vi "Send Host Stream Command Start.vi"(6 "Project Folder":path, 8 "error in (no error)":errorcluster, 9 "Addon":string, 10 "Target IP Address":string, 11 "Q Refs":T1) -> (0 "error out":errorcluster)   [LabVIEW 2019, in "CAN Stream Support Workspace Shared.lvlib"]
uses:
  CAN Stream Support Workspace Shared.lvlib
  Types/Host Stream Queue Refs.ctl
  Types/Host Stream Queue Type.ctl
  Types/Host Stream Queue Command.ctl
  <vilib>/xnet/xnet.llb/XNET Frame CAN.ctl
  <vilib>/xnet/xnet.llb/XNET Frame Type CAN.ctl
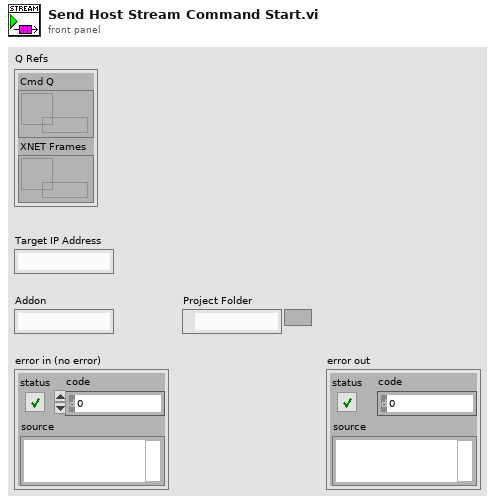
[diagram p1: front panel]
types:
  T1 = typedef "CAN Stream Support Workspace Shared.lvlib/Host Stream Queue Refs.ctl" = cluster{"Cmd Q":refnum<queue>, "XNET Frames":refnum<queue>}
  T2 = typedef "CAN Stream Support Workspace Shared.lvlib/Host Stream Queue Type.ctl" = cluster{"Cmd":T3, "Target IP Address":string, "Addon":string, "Project Folder":path}
  T3 = typedef "CAN Stream Support Workspace Shared.lvlib/Host Stream Queue Command.ctl" = enum8{"Start Stream", "Stop Stream", "Exit"}
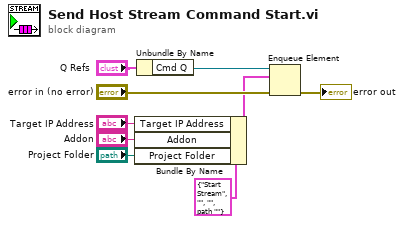
[diagram p0: block diagram]
diagram:
  n1 = Bundle By Name(cluster=T2 {"Cmd"=enum."Start Stream", "Target IP Address"="", "Addon"="", "Project Folder"=path ""} ("element"), "Target IP Address"="Target IP Address", "Addon"="Addon", "Project Folder"="Project Folder") -> (w5:T2)
  n2 = Unbundle By Name("Q Refs") -> ("Cmd Q"=w2:refnum<queue>)
  n3 = Enqueue Element(queue=w2, element=w5, error in (no error)="error in (no error)") -> (error out=→"error out":errorcluster)  [unwired: 1 in, 2 out]
